vi "Write INodeFactory.vi"(10 "INodeFactory":refnum<class "INodeFactory.lvclass">, 11 "Search in":refnum<class "Search.lvclass">) -> (3 "Search out":refnum<class "Search.lvclass">)   [LabVIEW 2016, in "Search.lvclass"]
uses:
  Search.lvclass
  INodeFactory/INodeFactory.lvclass
  Search.lvclass/Search.ctl
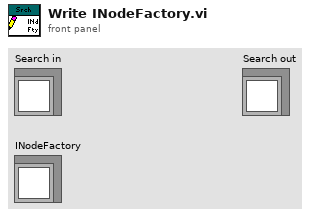
[diagram p1: front panel]
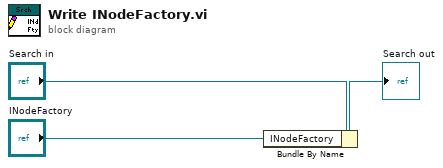
[diagram p0: block diagram]
diagram:
  n1 = Bundle By Name(cluster="Search in", "INodeFactory"="INodeFactory") -> (→"Search out":refnum<class "Search.lvclass">)
